vi "zlib Uncompress.vi"(8 "error in (no error)":errorcluster, 10 "Uncompressed Size in":u32, 11 "Compressed Data in":string) -> (0 "error out":errorcluster, 2 "Uncompressed Size out":i32, 3 "Uncompressed Data out":string)   [LabVIEW 2022 SP3, in "VI-Hacker.lvlib"]
doc: "zlib Deflate uncompression."
uses:
  VI-Hacker.lvlib
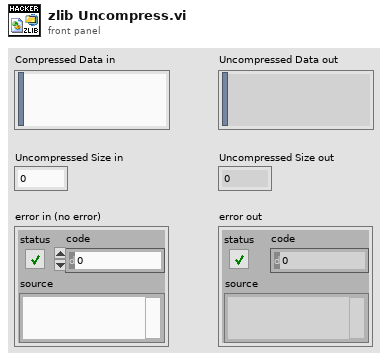
[diagram p1: front panel]
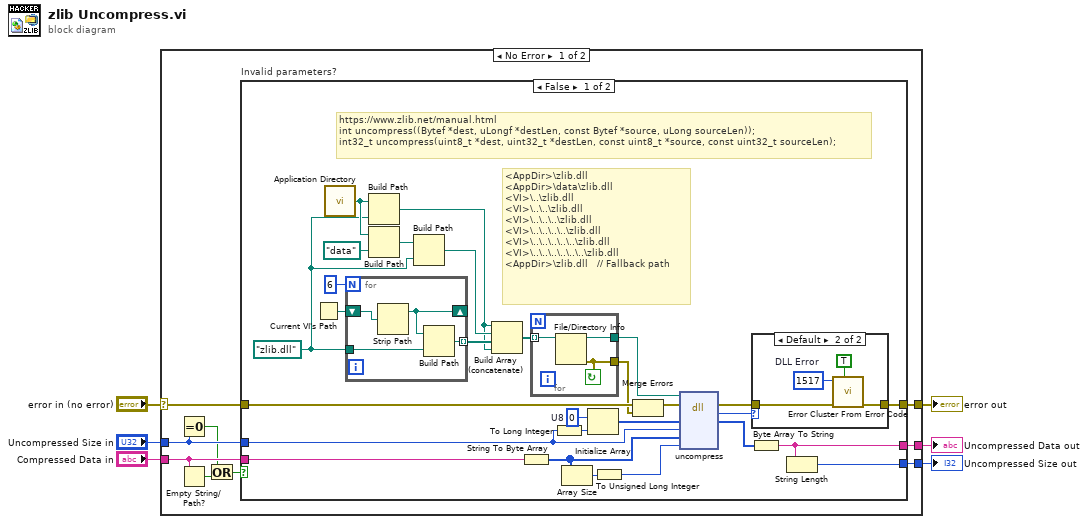
[diagram p0: block diagram]
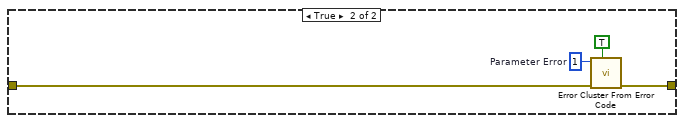
[diagram p3: hidden frame]
diagram:
  n1 = case shown="No Error" "error in (no error)" {
    selector: "error in (no error)" -> [w15 w60]
    tunnel: "Uncompressed Size in" -> [w12 _]
    tunnel: "Compressed Data in" -> [w11 _]
    tunnel: [w14 w60] -> w3
    tunnel: [w13 _] -> w2
    tunnel: [w7 _] -> w1
    frame No Error {
      n2 = Equal To 0?(x=w12) -> (x = 0?=w9:bool)
      n3 = Empty String/Path?(string/path=w11) -> (empty?=w10:bool)
      n4 = Or(x=w9, y=w10) -> (x .or. y?=w8:bool)
      n5 = case "Invalid parameters?" shown="False" w8 {
        tunnel: w15 -> [w19 w58]
        tunnel: w12 -> [w41 _]
        tunnel: w11 -> [w40 _]
        tunnel: [w33 w57] -> w14
        tunnel: [w31 _] -> w13
        tunnel: [w30 _] -> w7
        frame False {
          w22 = path "zlib.dll"
          w43 = u8 0  # U8
          # "https://www.zlib.net/manual.html\nint uncompress((Bytef *dest, uLongf *destLen, const Bytef *source, uLong sourceLen));\nint32_t uncompress(uint8_t *dest, uint32_t *destLen, const uint8_t *source, const uint32_t sourceLen);"
          # "<AppDir>\\zlib.dll\n<AppDir>\\data\\zlib.dll\n<VI>\\..\\zlib.dll\n<VI>\\..\\..\\zlib.dll\n<VI>\\..\\..\\..\\zlib.dll\n<VI>\\..\\..\\..\\..\\zlib.dll\n<VI>\\..\\..\\..\\..\\..\\zlib.dll\n<VI>\\..\\..\\..\\..\\..\\..\\zlib.dll\n<AppDir>\\zlib.dll   // Fallback path"
          n6 = Current VI's Path() -> (path=w24:path)
          n7 = call <vilib>:"Application Directory.vi"() -> ("Application Directory"=w28:path)
          n8 = for {
            N: 6 -> [_]
            shift-right: [w46] -> _
            shift-left: w24 -> [w47]
            tunnel: w22 -> [w45]
            tunnel: [w44] -> w21 mode=indexing
            n9 = Strip Path(path=w47) -> (stripped path=w46:path)  [unwired: 1 out]
            n10 = Build Path(base path=w46, name or relative path=w45) -> (appended path=w44:path)
          }
          n11 = Build Path(base path=w28, name or relative path=w22) -> (appended path=w20:path)
          n12 = Build Path(base path=w28, name or relative path=path "data") -> (appended path=w27:path)
          n13 = Build Path(base path=w27, name or relative path=w22) -> (appended path=w26:path)
          n14 = Build Array (concatenate)(w20, w26, w21, w20) -> (w25:path[])
          n15 = String To Byte Array(string=w40) -> (unsigned byte array=w37:u8[])
          n16 = for {
            tunnel: w25 -> [w50] mode=indexing
            tunnel: [w49] -> w17
            tunnel: [w48] -> w16
            stop <- w49 continue-if-true
            n17 = File/Directory Info(path=w50) -> (path out=w48:path, error out=w49:errorcluster)  [unwired: 1 in, 5 out]
          }
          n18 = To Long Integer(number=w41) -> (32bit integer=w38:i32)
          n19 = Array Size(array=w37) -> (size(s)=w36:i32)
          n20 = Initialize Array(w43, w38) -> (w42:u8[])
          n21 = To Unsigned Long Integer(number=w36) -> (unsigned 32bit integer=w39:u32)
          n22 = Merge Errors(w19, w17) -> (w18:errorcluster)
          n23 = dll-call lib="zlib.dll" fn="uncompress"(path in=w16, error in=w18, "dest"=w42, "destLen"=w41, "source"=w37, "sourceLen"=w39) -> (error out=w34:errorcluster, "return type"=w35:i32, "dest"=w32:u8[])  [unwired: 4 in, 1 out]
          n24 = Byte Array To String(unsigned byte array=w32) -> (string=w31:string)
          n25 = case shown="Default" w35 {
            tunnel: w34 -> [w51 w53]
            tunnel: [w51 w52] -> w33
            frame 0 {
            }
            frame Default {
              w55 = 1517  # DLL Error
              n26 = call <vilib>:"Error Cluster From Error Code.vi"("show call chain? (False)"=TRUE, "error in (no error)"=w53, "error code (0)"=w55) -> ("error out"=w52:errorcluster)  [unwired: 6 in]
            }
          }
          n27 = String Length(string=w31) -> (length=w30:i32)
        }
        frame True {
          w59 = 1  # Parameter Error
          n28 = call <vilib>:"Error Cluster From Error Code.vi"("show call chain? (False)"=TRUE, "error in (no error)"=w58, "error code (0)"=w59) -> ("error out"=w57:errorcluster)  [unwired: 6 in]
        }
      }
    }
    frame Error {
    }
  }
  "error out" <- w3
  "Uncompressed Data out" <- w2
  "Uncompressed Size out" <- w1
